vi "Get Cursor Position.vi"(8 "Screen Offset":T2, 9 "Text Offset":T1, 10 "Line Numbers in":refnum<vi>, 11 "String in":refnum<vi>) -> (2 "Autocomplete Position":T2)   [LabVIEW 2016, in "Code String.lvclass"]
doc: "Determines the <b>Cursor Position</b> in global screen coordinates of the edit cursor in <b>String</b>.\nLeft = (Number of visible characters before cursor * Character Width) + Screen Offset\nTop = (Number of visible lines before line * Character Height) + Screen Offset\n\nUses the following reference points:\n<b>Line Numbers</b> -- a listbox that is positionally aligned with <b>String</b> and has a value equal to the line in <b>String</b> at which the edit cursor is positioned. Uses to determine the number of visible lines.\n<b>Text Offset</b> -- the number of visible charcters before the cursor\n<b>Screen Offset</b> -- the offset in screen coordinates of the origin of <b>String</b>.\n\n--------------------\nCopyright (c) 2019 Analog Devices, Inc. All rights reserved.\n\nRedistribution and use in source and binary forms, with or without modification,\nare permitted provided that the following conditions are met:\n - Redistributions of source code must retain the above copyright notice, this\n list of conditions and the following disclaimer.\n - Redistributions in binary form must reproduce the above copyright notice,\n this list of conditions and the following disclaimer in the documentation\n and/or other materials provided with the distribution.\n - Modified versions of the software must be conspicuously marked as such.\n - This software is licensed solely and exclusively for use with\n processors/products manufactured by or for Analog Devices, Inc.\n - This software may not be combined or merged with other code in any manner\n that would cause the software to become subject to terms and conditions\n which differ from those listed here.\n - Neither the name of Analog Devices, Inc. nor the names of its contributors\n may be used to endorse or promote products derived from this software\n without specific prior written permission.\n - The use of this software may or may not infringe the patent rights of one or\n more patent holders. This license does not release you from the requirement\n that you obtain separate licenses from these patent holders to use this\n software.\n\nTHIS SOFTWARE IS PROVIDED BY ANALOG DEVICES, INC. AND CONTRIBUTORS \"AS IS\" AND\nANY EXPRESS OR IMPLIED WARRANTIES, INCLUDING, BUT NOT LIMITED TO,\nNON-INFRINGEMENT, TITLE, MERCHANTABILITY AND FITNESS FOR A PARTICULAR PURPOSE\nARE DISCLAIMED. IN NO EVENT SHALL ANALOG DEVICES, INC. OR CONTRIBUTORS BE LIABLE\nFOR ANY DIRECT, INDIRECT, INCIDENTAL, SPECIAL, EXEMPLARY, PUNITIVE OR\nCONSEQUENTIAL DAMAGES (INCLUDING, BUT NOT LIMITED TO, DAMAGES ARISING OUT OF\nCLAIMS OF INTELLECTUAL PROPERTY RIGHTS INFRINGEMENT; PROCUREMENT OF SUBSTITUTE\nGOODS OR SERVICES; LOSS OF USE, DATA, OR PROFITS; OR BUSINESS INTERRUPTION)\nHOWEVER CAUSED AND ON ANY THEORY OF LIABILITY, WHETHER IN CONTRACT, STRICT\nLIABILITY, OR TORT (INCLUDING NEGLIGENCE OR OTHERWISE) ARISING IN ANY WAY OUT OF\nTHE USE OF THIS SOFTWARE, EVEN IF ADVISED OF THE POSSIBILITY OF SUCH DAMAGE.\n\n2019-01-10-7CBSD SLA"
uses:
  Code String.lvclass
  <vilib>/Utility/miscctls.llb/LVPositionTypeDef.ctl
  <vilib>/Utility/miscctls.llb/LVSelectionTypeDef.ctl
panel:
  # "Copyright (c) 2019 Analog Devices, Inc.  All rights reserved.\n\nRedistribution and use in source and binary forms, with or without modification,\nare permitted provided that the following conditions are met:\n  - Redistributions of source code must retain the above copyright notice, this\n    list of conditions and the following disclaimer.\n  - Redistributions in binary form must reproduce the above copyright notice,\n    this list of conditions and the following disclaimer in the documentation\n    and/or other materials provided with the distribution.\n  - Modified versions of the software must be conspicuously marked as such.\n  - This software is licensed solely and exclusively for use with\n    processors/products manufactured by or for Analog Devices, Inc.\n  - This software may not be combined or merged with other code in any manner\n    that would cause the software to become subject to terms and conditions\n    which differ from those listed here.\n  - Neither the name of Analog Devices, Inc. nor the names of its contributors\n    may be used to endorse or promote products derived from this software\n    without specific prior written permission.\n  - The use of this software may or may not infringe the patent rights of one or\n    more patent holders.  This license does not release you from the requirement\n    that you obtain separate licenses from these patent holders to use this\n    software.\n\nTHIS SOFTWARE IS PROVIDED BY ANALOG DEVICES, INC. AND CONTRIBUTORS \"AS IS\" AND\nANY EXPRESS OR IMPLIED WARRANTIES, INCLUDING, BUT NOT LIMITED TO,\nNON-INFRINGEMENT, TITLE, MERCHANTABILITY AND FITNESS FOR A PARTICULAR PURPOSE\nARE DISCLAIMED. IN NO EVENT SHALL ANALOG DEVICES, INC. OR CONTRIBUTORS BE LIABLE\nFOR ANY DIRECT, INDIRECT, INCIDENTAL, SPECIAL, EXEMPLARY, PUNITIVE OR\nCONSEQUENTIAL DAMAGES (INCLUDING, BUT NOT LIMITED TO, DAMAGES ARISING OUT OF\nCLAIMS OF INTELLECTUAL PROPERTY RIGHTS INFRINGEMENT; PROCUREMENT OF SUBSTITUTE\nGOODS OR SERVICES; LOSS OF USE, DATA, OR PROFITS; OR BUSINESS INTERRUPTION)\nHOWEVER CAUSED AND ON ANY THEORY OF LIABILITY, WHETHER IN CONTRACT, STRICT\nLIABILITY, OR TORT (INCLUDING NEGLIGENCE OR OTHERWISE) ARISING IN ANY WAY OUT OF\nTHE USE OF THIS SOFTWARE, EVEN IF ADVISED OF THE POSSIBILITY OF SUCH DAMAGE.\n\n2019-01-10-7CBSD SLA"
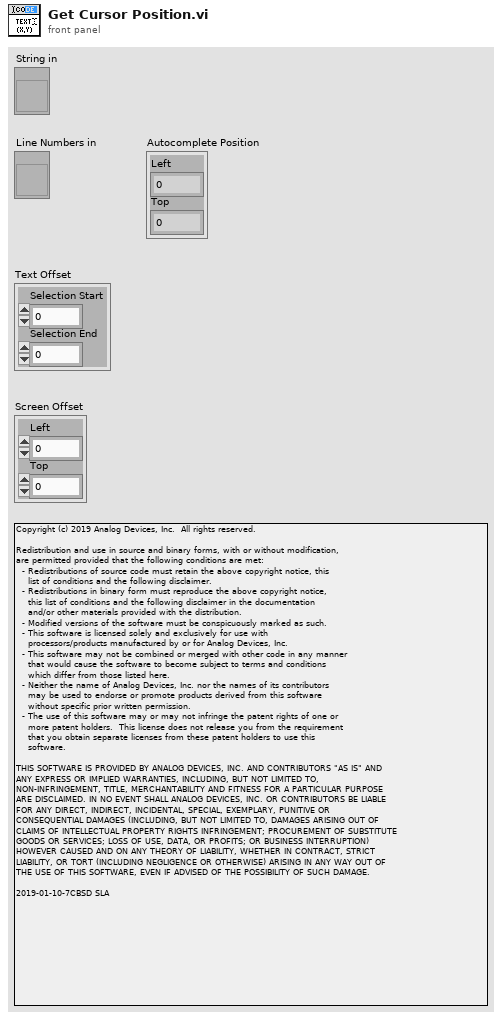
[diagram p1: front panel]
types:
  T1 = typedef "LVSelectionTypeDef.ctl" = cluster{"Selection Start":u32, "Selection End":u32}
  T2 = typedef "LVPositionTypeDef.ctl" = cluster{"Left":i32, "Top":i32}
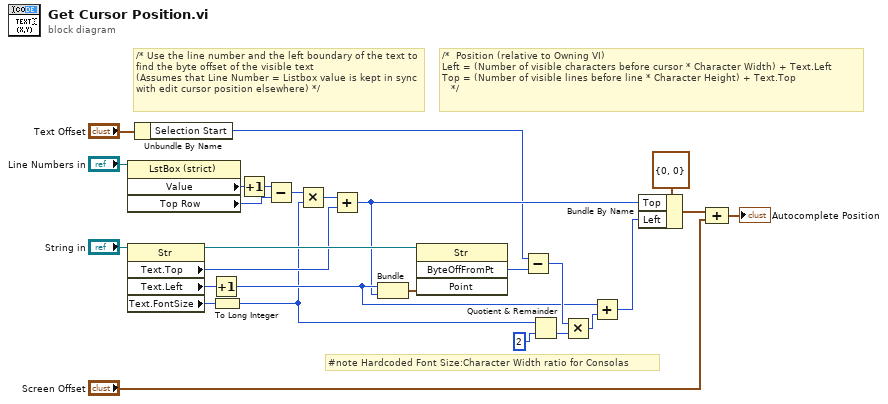
[diagram p0: block diagram]
diagram:
  # "#note Hardcoded Font Size:Character Width ratio for Consolas"
  # "/*  Position (relative to Owning VI)\nLeft = (Number of visible characters before cursor * Character Width) + Text.Left\nTop = (Number of visible lines before line * Character Height) + Text.Top\n   */"
  # "/* Use the line number and the left boundary of the text to find the byte offset of the visible text\n(Assumes that Line Number = Listbox value is kept in sync with edit cursor position elsewhere) */"
  n1 = property on="Property Node" class="LstBox (strict)"(reference="Line Numbers in") -> ("Value"=w7:i32, "Top Row"=w18:i32)  [unwired: 1 in, 2 out]
  n2 = property on="Property Node" class="Str"(reference="String in") -> (reference out=w15:refnum<vi>, "Text.Top"=w9:i32, "Text.Left"=w10:i32, "Text.FontSize"=w16:u32)  [unwired: 1 in, 1 out]
  n3 = Unbundle By Name("Text Offset") -> ("Selection Start"=w3:u32)
  n4 = Increment(x=w10) -> (x+1=w11:i32)
  n5 = To Long Integer(number=w16) -> (32bit integer=w8:i32)
  n6 = Increment(x=w7) -> (x+1=w4:i32)
  n7 = Subtract(x=w4, y=w18) -> (x-y=w6:i32)
  n8 = Multiply(x=w6, y=w8) -> (x*y=w17:i32)
  n9 = Add(x=w17, y=w9) -> (x+y=w5:i32)
  n10 = Bundle(w11, w5) -> (w24:cluster{i32, i32})  [unwired: 1 in]
  n11 = invoke on="Invoke Node" class="Str" method="ByteOffFromPt"(reference=w15, "Point"=w24) -> ("ByteOffFromPt"=w12:i32)  [unwired: 2 in, 3 out]
  n12 = Subtract(x=w3, y=w12) -> (x-y=w19:u32)
  n13 = Quotient & Remainder(x=w8, y=2 ("x")) -> (floor(x/y)=w20:i32)  [unwired: 1 out]
  n14 = Multiply(x=w19, y=w20) -> (x*y=w22:u32)
  n15 = Add(x=w11, y=w22) -> (x+y=w14:u32)
  n16 = Bundle By Name(cluster=T2 {"Left"=0, "Top"=0} ("Position"), "Top"=w5, "Left"=w14) -> (w13:T2)
  n17 = Compound Arithmetic op=ADD(w13, "Screen Offset") -> (→"Autocomplete Position":T2)
